vi "Read or Write Configurations.vi"(0 "Architecture":string, 5 "Maintainer":string, 7 "Email":string, 11 "error in (no error)":errorcluster, 13 "Operation":T1) -> (4 "Architecture OUT":string, 6 "Maintainer OUT":string, 8 "Email OUT":string, 15 "error out":errorcluster)   [LabVIEW 2021, in "Measurement Builder.lvlib"]
uses:
  Measurement Builder.lvlib
  controls/Config File Operations.ctl
  <vilib>/Utility/config.llb/Read Key (String).vi
  <vilib>/Utility/config.llb/Write Key (String).vi
  <vilib>/Utility/config.llb/NI_LVConfig.lvlib
  Path Functions/Path Functions.lvlib
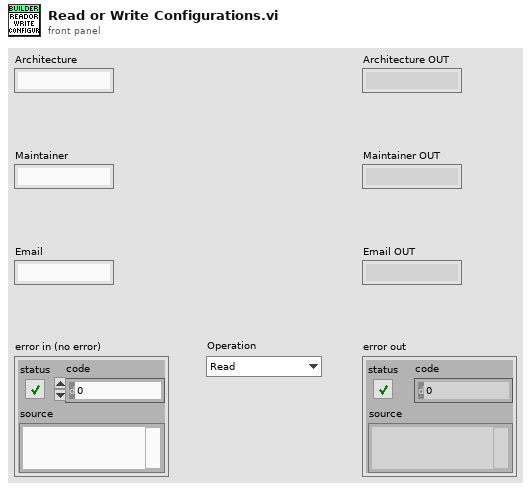
[diagram p1: front panel]
types:
  T1 = typedef "Measurement Builder.lvlib/Config File Operations.ctl" = enum16{"Read", "Write"}
  T2 = typedef "NI_LVConfig.lvlib/Config Data RefNum.ctl" = refnum<k1>
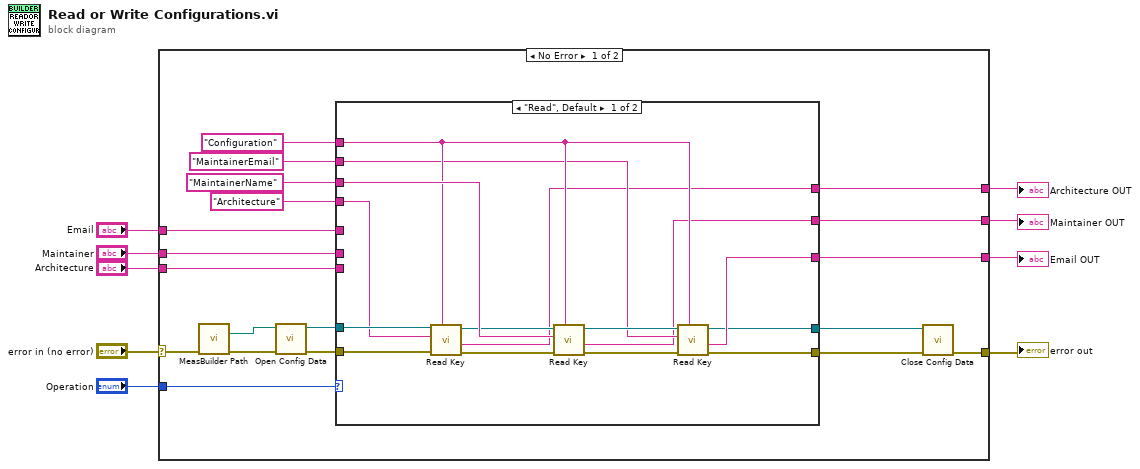
[diagram p0: block diagram]
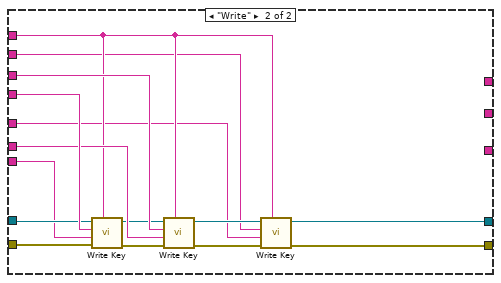
[diagram p2: hidden frame]
diagram:
  n1 = case shown="No Error" "error in (no error)" {
    selector: "error in (no error)" -> [w28 w59]
    tunnel: "Operation" -> [w22 _]
    tunnel: [w16 w59] -> w7
    tunnel: [w15 _] -> w6
    tunnel: [w14 _] -> w5
    tunnel: [w13 _] -> w4
    tunnel: "Architecture" -> [w12 _]
    tunnel: "Maintainer" -> [w11 _]
    tunnel: "Email" -> [w10 _]
    frame No Error {
      n2 = call "MeasBuilder Path.vi"("error in (no error)"=w28) -> ("Config"=w26:path, "error out"=w27:errorcluster)  [unwired: 11 in, 2 out]
      n3 = call <vilib>:"Open Config Data.vi"("error in (no error)"=w27, "configuration file path"=w26) -> ("error out"=w25:errorcluster, "refnum"=w24:T2)  [unwired: 7 in, 1 out]
      n4 = case shown="\"Read\", Default" w22 {
        tunnel: w25 -> [w43 w49]
        tunnel: w24 -> [w42 w57]
        tunnel: "Configuration" ("section") -> [w38 w53]
        tunnel: "Architecture" ("section") -> [w41 w58]
        tunnel: "MaintainerName" ("section") -> [w39 w55]
        tunnel: "MaintainerEmail" ("section") -> [w35 w46]
        tunnel: [w33 w51] -> w18
        tunnel: [w32 _] -> w13
        tunnel: [w31 _] -> w14
        tunnel: [w30 _] -> w15
        tunnel: [w29 w52] -> w17
        tunnel: w12 -> [_ w56]
        tunnel: w11 -> [_ w54]
        tunnel: w10 -> [_ w45]
        frame "Read", Default {
          n5 = call-poly <vilib>:"Read Key.vi"("section"=w38, "error in (no error)"=w43, "key"=w41, "refnum"=w42) -> ("error out"=w40:errorcluster, "value"=w30:string, "refnum out"=w36:T2)  [unwired: 4 in, 1 out]
          n6 = call-poly <vilib>:"Read Key.vi"("section"=w38, "error in (no error)"=w40, "key"=w39, "refnum"=w36) -> ("error out"=w34:errorcluster, "value"=w31:string, "refnum out"=w37:T2)  [unwired: 4 in, 1 out]
          n7 = call-poly <vilib>:"Read Key.vi"("section"=w38, "error in (no error)"=w34, "key"=w35, "refnum"=w37) -> ("error out"=w33:errorcluster, "value"=w32:string, "refnum out"=w29:T2)  [unwired: 4 in, 1 out]
        }
        frame "Write" {
          n8 = call-poly <vilib>:"Write Key.vi"("section"=w53, "error in (no error)"=w49, "value"=w56, "key"=w58, "refnum"=w57) -> ("error out"=w48:errorcluster, "refnum out"=w44:T2)  [unwired: 4 in, 1 out]
          n9 = call-poly <vilib>:"Write Key.vi"("section"=w53, "error in (no error)"=w48, "value"=w54, "key"=w55, "refnum"=w44) -> ("error out"=w50:errorcluster, "refnum out"=w47:T2)  [unwired: 4 in, 1 out]
          n10 = call-poly <vilib>:"Write Key.vi"("section"=w53, "error in (no error)"=w50, "value"=w45, "key"=w46, "refnum"=w47) -> ("error out"=w51:errorcluster, "refnum out"=w52:T2)  [unwired: 4 in, 1 out]
        }
      }
      n11 = call <vilib>:"Close Config Data.vi"("error in (no error)"=w18, "refnum"=w17) -> ("error out"=w16:errorcluster)  [unwired: 8 in, 1 out]
    }
    frame Error {
    }
  }
  "error out" <- w7
  "Email OUT" <- w4
  "Maintainer OUT" <- w5
  "Architecture OUT" <- w6
